vi "Manager.vi"() -> ()   [LabVIEW 2021, in "CIFPluginManager.lvclass"]
uses:
  CIFPluginManager.lvclass
  CIFPluginManager.lvclass/CIFPluginManager.ctl
  <vilib>/gRPC/LabVIEW gRPC Servicer/Servicer/Servicer.lvclass
  gRPC/CIF_Manager_server/RPC Service/Manager/Manager.lvclass
  CIFUtilities/CIFLogs/CIFLogs.lvlib
  gRPC/CIF_Manager_client/RPC Messages/cif_common_Empty.ctl
  gRPC/CIF_Manager_client/CIF_Manager_client.lvlib
  <vilib>/Utility/miscctls.llb/LVMapReplaceAction.ctl
  CIFCore/Grpc/CIFCoreWrapper/CIFCoreWrapper.lvlib
  CIFUtilities/CIFConfigurationFile/CIF Configuration File.lvlib
  gRPC/CIF_Manager_server/RPC Messages/cif_manager_ErrorInfo.ctl
  gRPC/CIF_Manager_server/CIF_Manager_server.lvlib
  gRPC/CIF_Manager_server/RPC Messages/cif_manager_ErrorInfoList.ctl
  gRPC/CIF_Manager_server/RPC Messages/cif_manager_FileData.ctl
  gRPC/CIF_Manager_server/RPC Messages/cif_manager_PluginInfo.ctl
  gRPC/CIF_Manager_server/RPC Messages/cif_manager_PluginInfoArray.ctl
  gRPC/CIF_Manager_server/RPC Messages/cif_manager_PluginType.ctl
  gRPC/CIF_Manager_server/RPC Messages/cif_manager_PluginTypeReply.ctl
  gRPC/CIF_Manager_server/RPC Messages/cif_manager_PluginInfoResponse.ctl
  CIFCore/Common/CIFCoreCommon.lvlib
  CIFCore/Common/Typedef/Errors.ctl
  gRPC/CIF_Manager_server/RPC Messages/cif_manager_TimePair.ctl
  gRPC/CIF_Manager_server/RPC Messages/cif_manager_ClockConversion.ctl
  gRPC/CIF_Manager_server/RPC Messages/cif_manager_ClockConversionArray.ctl
  gRPC/CIF_Manager_server/RPC Messages/cif_manager_SystemStatus.ctl
  gRPC/CIF_Manager_server/RPC Messages/cif_manager_OrchReturn.ctl
  CIFUtilities/Scripting/Orchestration/Python/Python Orchestration.lvlib
  <vilib>/CIF Foundation/CIF Utilities/Time/Time_CIF_U.lvlib
  <vilib>/CIF Foundation/CIF Utilities/Time/Typedef/Timestamp Pair.ctl
  gRPC/CIF_Manager_server/RPC Messages/cif_common_ShortVersion.ctl
  gRPC/CIF_Manager_server/RPC Messages/cif_common_Status.ctl
  gRPC/CIF_Manager_server/RPC Messages/cif_plugincore_MonitorI64.ctl
  gRPC/CIF_Manager_server/RPC Messages/cif_plugincore_MonitorU64.ctl
  gRPC/CIF_Manager_server/RPC Messages/cif_plugincore_MonitorDoubles.ctl
  gRPC/CIF_Manager_server/RPC Messages/cif_plugincore_Error.ctl
  gRPC/CIF_Manager_server/RPC Messages/cif_common_TimingStats.ctl
  gRPC/CIF_Manager_server/RPC Messages/cif_plugincore_FifoStatistics.ctl
  gRPC/CIF_Manager_server/RPC Messages/cif_plugincore_TimingStatistics.ctl
  gRPC/CIF_Manager_server/RPC Messages/cif_plugincore_StatusData_State.ctl
  gRPC/CIF_Manager_server/RPC Messages/cif_plugincore_StatusData.ctl
panel:
  out "error out":errorcluster
  in  "stop":bool
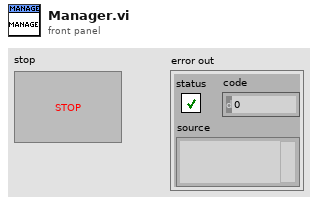
[diagram p1: front panel]
types:
  T1 = typedef "CIF_Manager_client.lvlib/cif_common_Empty.ctl" = cluster{"void":string}
  T2 = typedef "LVMapReplaceAction.ctl" = enum32{"Modify Entry only if found", "Add or Modify Entry", "Delete Entry"}
  T3 = typedef "CIF_Manager_server.lvlib/cif_manager_PluginTypeReply.ctl" = cluster{"plugin_types":T4[]}
  T4 = typedef "CIF_Manager_server.lvlib/cif_manager_PluginType.ctl" = cluster{"plugin_type":string, "plugin_version":T5}
  T5 = typedef "CIF_Manager_server.lvlib/cif_common_ShortVersion.ctl" = cluster{"major":u32, "minor":u32, "fix":u32}
  T6 = typedef "CIF_Manager_server.lvlib/cif_manager_ErrorInfoList.ctl" = cluster{"error_info":T7[]}
  T7 = typedef "CIF_Manager_server.lvlib/cif_manager_ErrorInfo.ctl" = cluster{"error_status":bool, "error_code":i32, "plugin":string, "time":string, "message":string, "location":string}
  T8 = typedef "CIF_Manager_server.lvlib/cif_manager_FileData.ctl" = cluster{"data":string}
  T9 = typedef "CIF_Manager_server.lvlib/cif_manager_PluginInfoArray.ctl" = cluster{"plugin_info":T10[]}
  T10 = typedef "CIF_Manager_server.lvlib/cif_manager_PluginInfo.ctl" = cluster{"plugin_name":string, "plugin_type":string, "grpc_port":i32, "plugin_version":T5, "status":T11}
  T11 = typedef "CIF_Manager_server.lvlib/cif_plugincore_StatusData.ctl" = cluster{"state":T12, "timing_statistics":T13, "fifo_statistics":T15, "error":T16, "monitor_doubles":T17, "monitor_u64s":T18, "monitor_i64s":T19}
  T12 = typedef "CIF_Manager_server.lvlib/cif_plugincore_StatusData_State.ctl" = enum32{"NULL", "CREATING", "LISTENING", "RUNNING", "CLEANINGUP", "DESTROYING"}
  T13 = typedef "CIF_Manager_server.lvlib/cif_plugincore_TimingStatistics.ctl" = cluster{"period":T14, "wake_error":T14, "execute":T14, "housekeep":T14, "idle":T14, "cleanup":T14, "custom_1":T14, "custom_2":T14}
  T14 = typedef "CIF_Manager_server.lvlib/cif_common_TimingStats.ctl" = cluster{"max":i64, "min":i64, "avg":dbl}
  T15 = typedef "CIF_Manager_server.lvlib/cif_plugincore_FifoStatistics.ctl" = cluster{"from_t0":T14, "from_previous_plugin":T14, "output_error":T14}
  T16 = typedef "CIF_Manager_server.lvlib/cif_plugincore_Error.ctl" = cluster{"status":bool, "code":i32}
  T17 = typedef "CIF_Manager_server.lvlib/cif_plugincore_MonitorDoubles.ctl" = cluster{"double_1":dbl, "double_2":dbl, "double_3":dbl, "double_4":dbl}
  T18 = typedef "CIF_Manager_server.lvlib/cif_plugincore_MonitorU64.ctl" = cluster{"u64_1":u64, "u64_2":u64, "u64_3":u64, "u64_4":u64}
  T19 = typedef "CIF_Manager_server.lvlib/cif_plugincore_MonitorI64.ctl" = cluster{"i64_1":i64, "i64_2":i64, "i64_3":i64, "i64_4":i64}
  T20 = typedef "CIFCoreCommon.lvlib/Errors.ctl" = enum16{"Invalid Clock ID", "Long Sleep", "gRPC Server Not Found", "Config Parse", "Timestamp Wrap", "Delayed Execution", "Duplicate Channel", "Missing Channel", "Incorrect Type", "Flatten Error", "Unflatten Data", "Unique Name", "Plugin Not Found", "Plugin Type Not Found", "Plugin Version Not Found", "Manager Not Found", "Numerical Issue", "Time Jump", "Clock ID Match", "Channel Length", "Plugin Connection", "gRPC Server Connection", "PPL Name Match", "Build", "Config Log Parse"}
  T21 = typedef "CIF_Manager_server.lvlib/cif_manager_PluginInfoResponse.ctl" = cluster{"plugin_info":T10, "status":T22}
  T22 = typedef "CIF_Manager_server.lvlib/cif_common_Status.ctl" = cluster{"code":i32, "message":string}
  T23 = typedef "CIF_Manager_server.lvlib/cif_manager_SystemStatus.ctl" = cluster{"clock_conversion_array":T24}
  T24 = typedef "CIF_Manager_server.lvlib/cif_manager_ClockConversionArray.ctl" = cluster{"clock_conversions":T25[]}
  T25 = typedef "CIF_Manager_server.lvlib/cif_manager_ClockConversion.ctl" = cluster{"clock_id":u32, "last_reset":u64, "slope":dbl, "offset_pair":T26, "clock_name":string}
  T26 = typedef "CIF_Manager_server.lvlib/cif_manager_TimePair.ctl" = cluster{"system_time":i64, "external_time":i64}
  T27 = typedef "Time_CIF_U.lvlib/Timestamp Pair.ctl" = cluster{"System Time":i64, "External Time":i64}
  T28 = typedef "CIF_Manager_server.lvlib/cif_manager_OrchReturn.ctl" = cluster{"orchestration_script":string, "status":T22}
  T29 = typedef "grpc-lvsupport-release.lvlib/grpcId.ctl" = u64
  T30 = typedef "CIF_Manager_server.lvlib/cif_manager_PluginConfig.ctl" = cluster{"plugin_type":string, "plugin_name":string, "version":string}
  T31 = typedef "CIF_Manager_client.lvlib/cif_common_Status.ctl" = cluster{"code":i32, "message":string}
  T32 = typedef "CIF_Manager_server.lvlib/cif_manager_RegisterData.ctl" = cluster{"plugin_name":string, "grpc_port":i32, "plugin_version":T5}
  T33 = typedef "CIFPluginManager.lvclass/Plugin Management Data.ctl" = cluster{"vi reference":refnum<vi>, "gRPC ID":T29, "Plugin Type":string, "Unique Name":string, "gRPC Port":i32, "Version":T34, "Load Timestamp":i64, "Unload Timestamp":i64, "Unloading":bool, "Ready for removal":bool, "status":T11}
  T34 = typedef "CIFCoreCommon.lvlib/Version.ctl" = cluster{"Major":i32, "Minor":i32, "Fix":i32, "Build":i32}
  T35 = typedef "CIF_Manager_server.lvlib/cif_manager_PluginName.ctl" = cluster{"plugin_name":string}
  T36 = typedef "CIFPluginManager.lvclass/Discovered Plugin.ctl" = cluster{"Filename":string, "Plugin Type":string, "Qualified name":string, "Version":T34}
  T37 = typedef "CIF_Manager_server.lvlib/cif_manager_QuerySettings.ctl" = cluster{"query_all":bool}
  T38 = typedef "CIFLogs.lvlib/Error Message.ctl" = cluster{"error":bool, "code":i32, "Message":string, "Location":string, "Plugin":string, "Time":string}
  T39 = typedef "CIF_Manager_server.lvlib/cif_manager_PluginStatus.ctl" = cluster{"pluginname":T35, "status":T11}
  T40 = typedef "Time_CIF_U.lvlib/Clock History Map.ctl" = map{u8, T41}
  T41 = typedef "Time_CIF_U.lvlib/Clock History.ctl" = cluster{"System Clock":i64[], "External Clock":i64[], "Last Reset Time":i64, "Slope":dbl[], "slope":dbl, "1/slope":dbl, "Offset Pair":T27, "Name":string}
  T42 = typedef "Time_CIF_U.lvlib/Clock Conversion.ctl" = cluster{"ClockID":u8, "Last Reset":i64, "Offset Pair":T27, "Slope":dbl, "1/Slope":dbl, "Name":string}
  T43 = typedef "CIF_Manager_server.lvlib/cif_manager_ClockUpdate.ctl" = cluster{"clock_id":u32, "timestamp_pair":T26, "reinit":bool, "clock_name":string}
  T44 = typedef "CIF_Manager_server.lvlib/cif_manager_OrchConfig.ctl" = cluster{"start_timestamp":u64, "create_file":bool, "orchestration_language":T45, "filename":string, "default_ip":string}
  T45 = typedef "CIF_Manager_server.lvlib/cif_manager_OrchestrationLanguage.ctl" = enum32{"NULL", "PYTHON"}
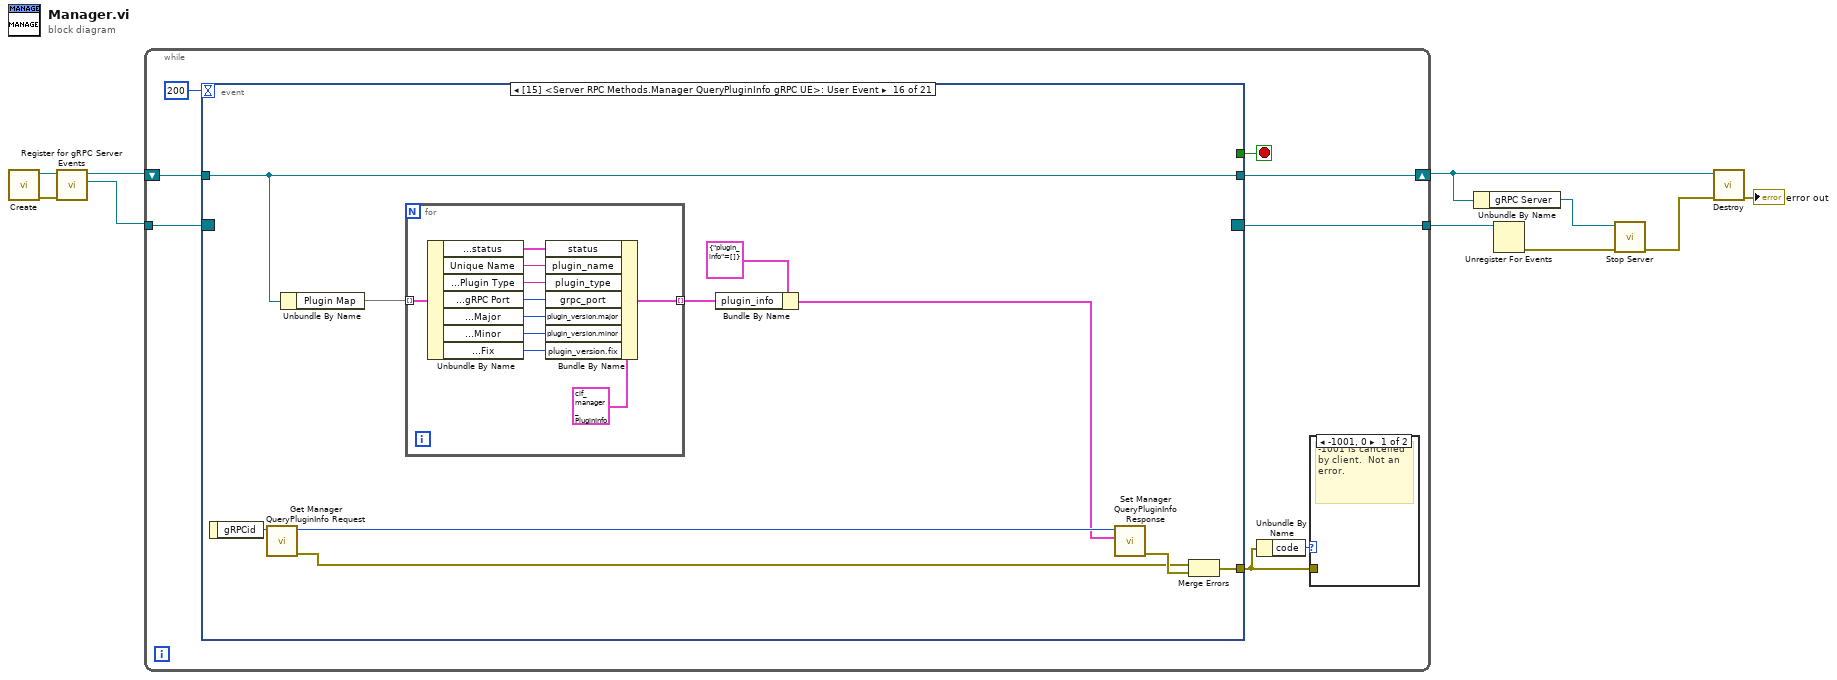
[diagram p0: block diagram]
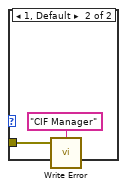
[diagram p2: hidden frame]
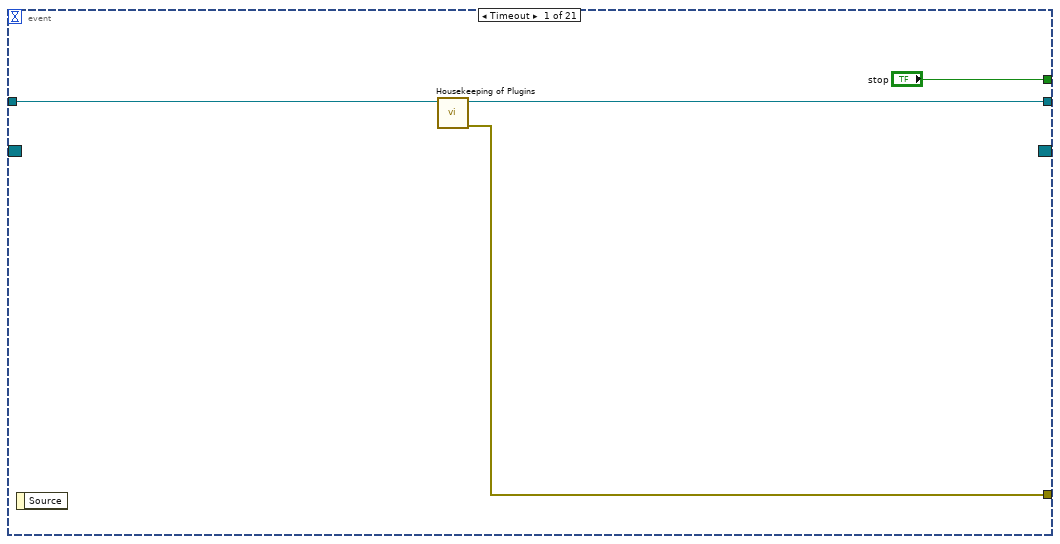
[diagram p3: hidden frame]
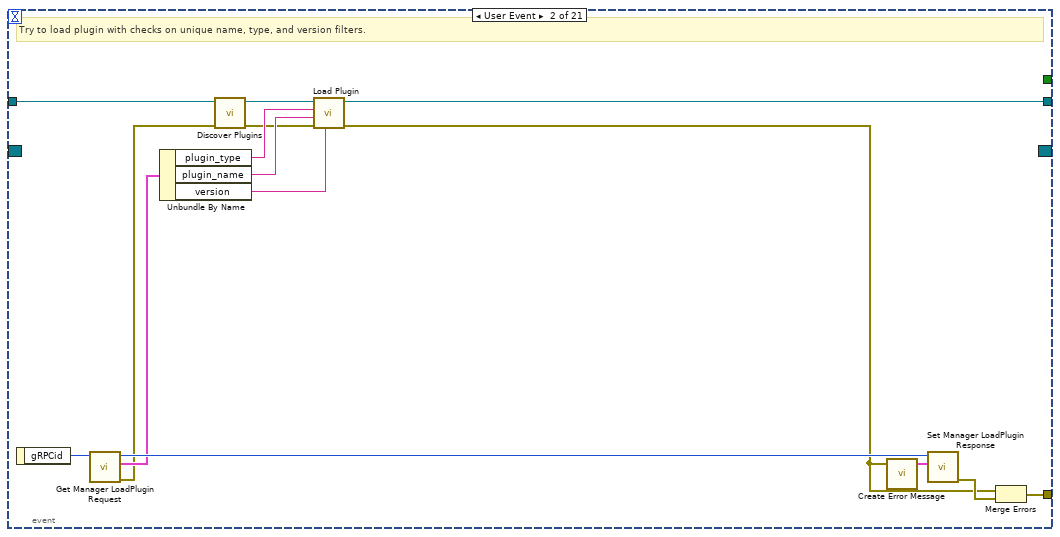
[diagram p4: hidden frame]
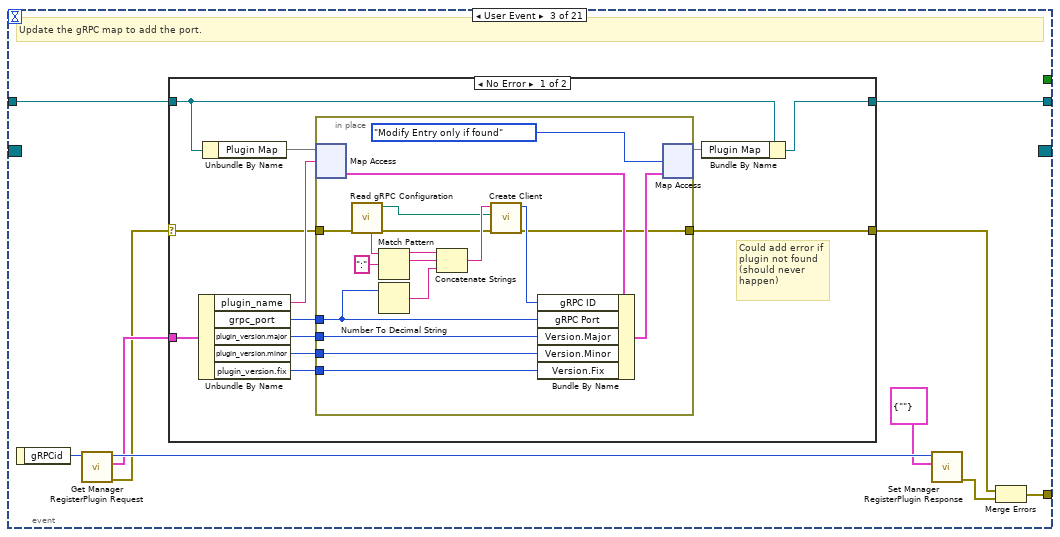
[diagram p5: hidden frame]
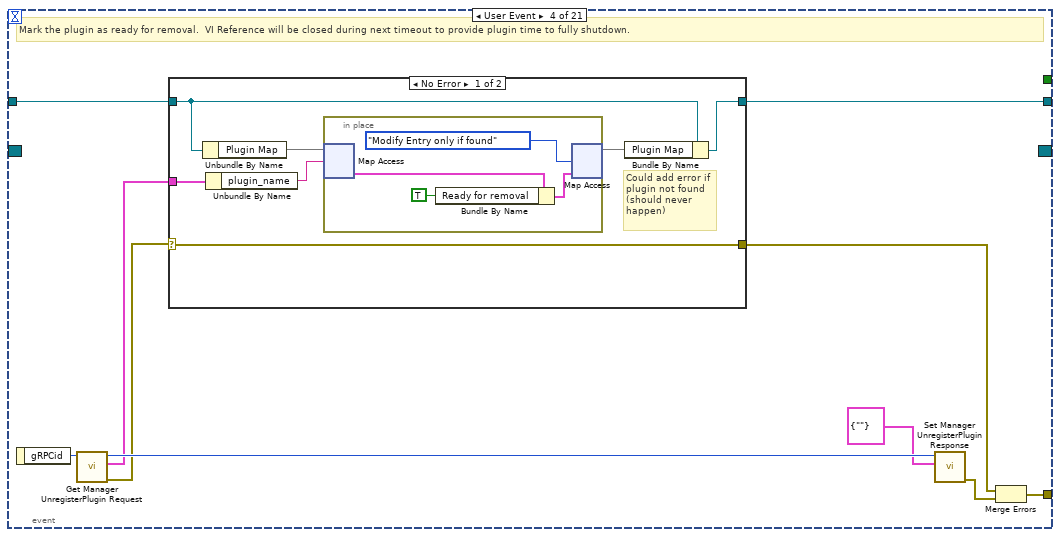
[diagram p7: hidden frame]
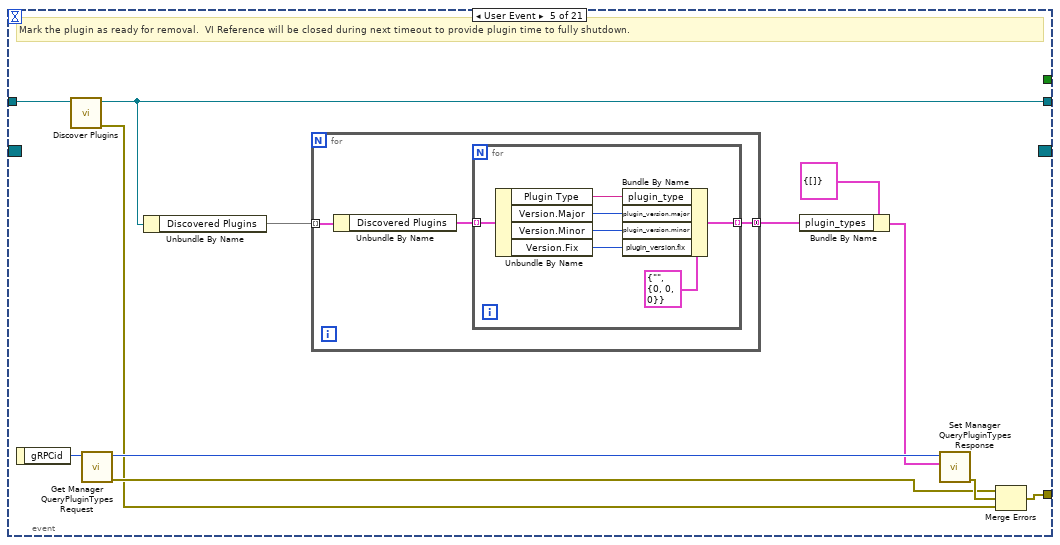
[diagram p9: hidden frame]
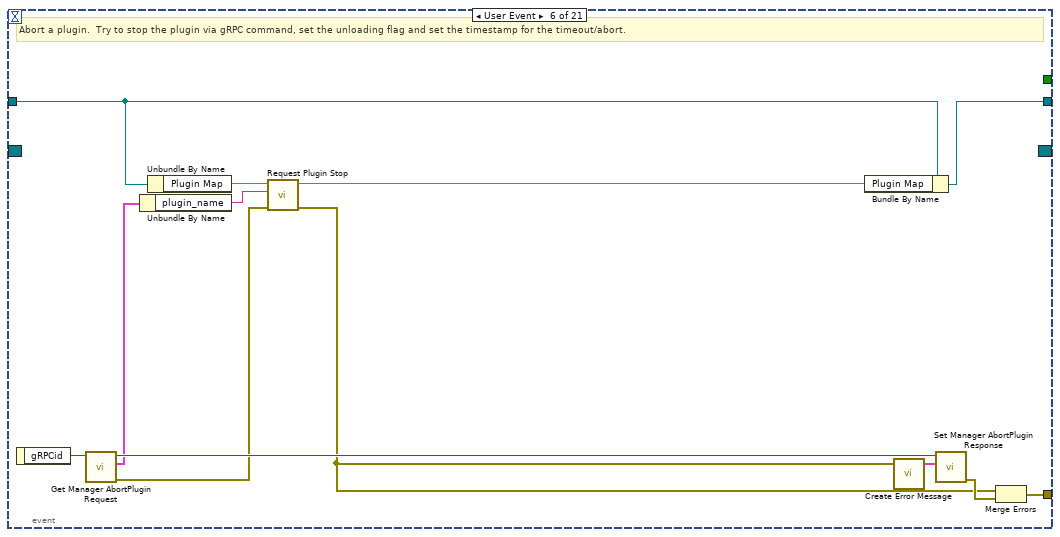
[diagram p10: hidden frame]
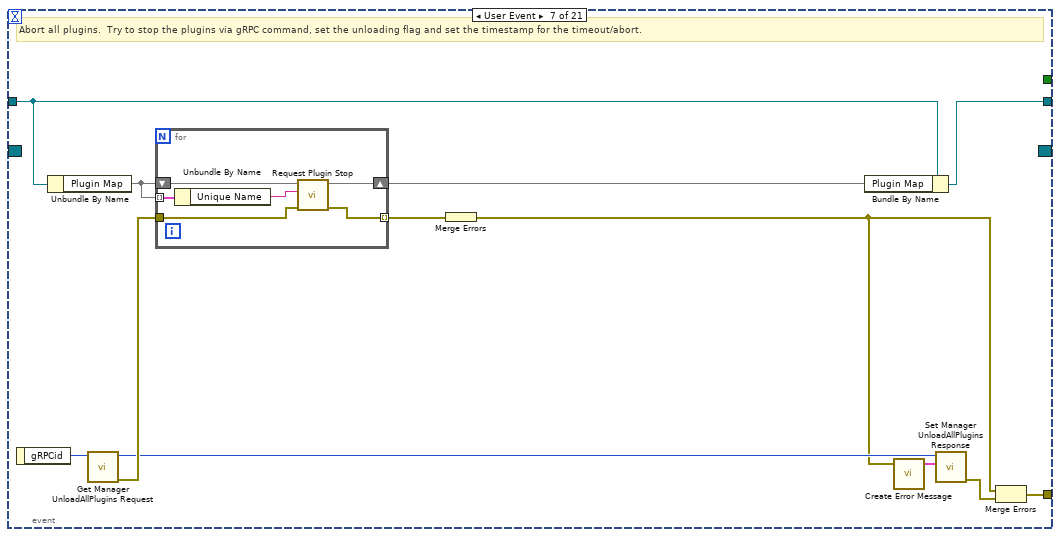
[diagram p11: hidden frame]
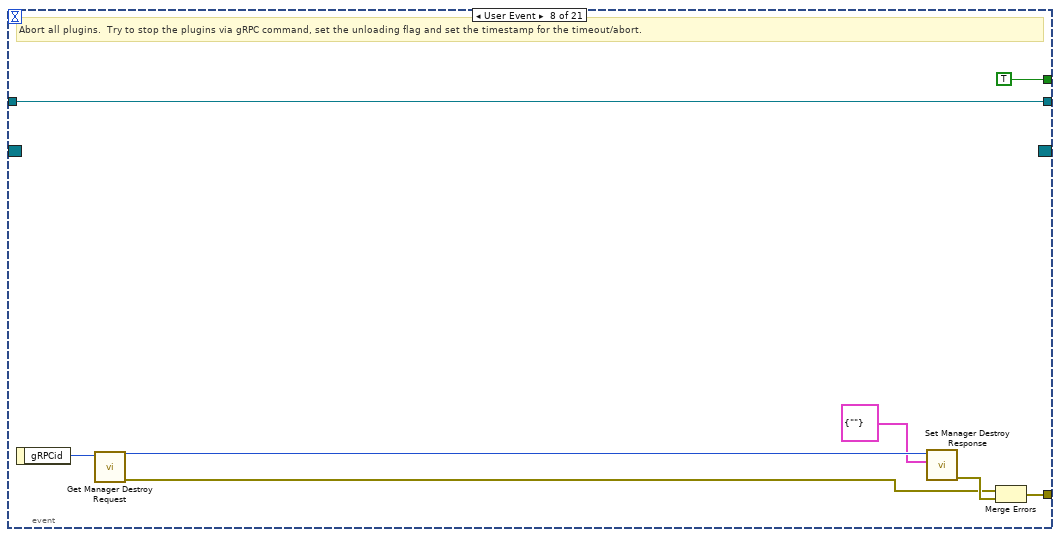
[diagram p12: hidden frame]
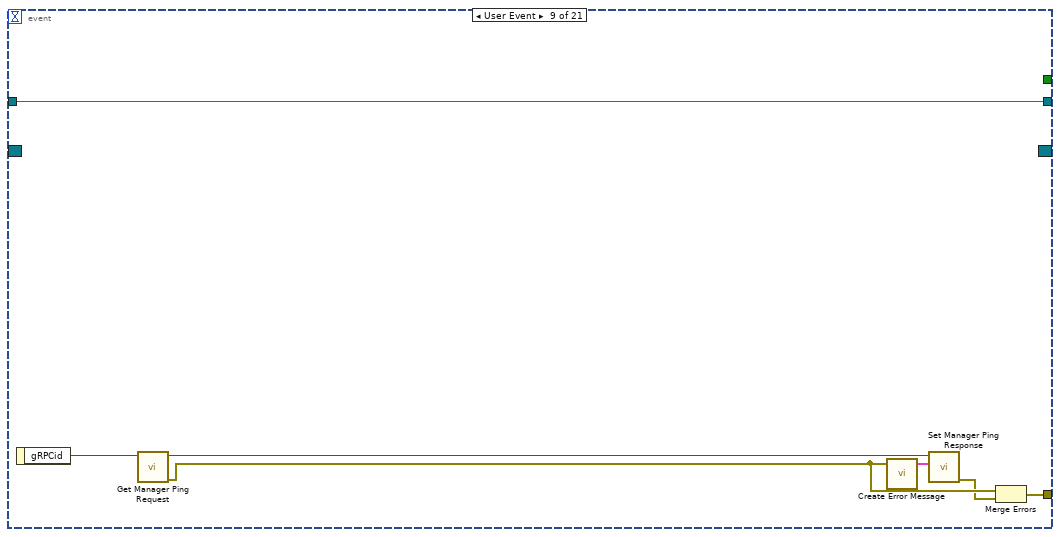
[diagram p13: hidden frame]
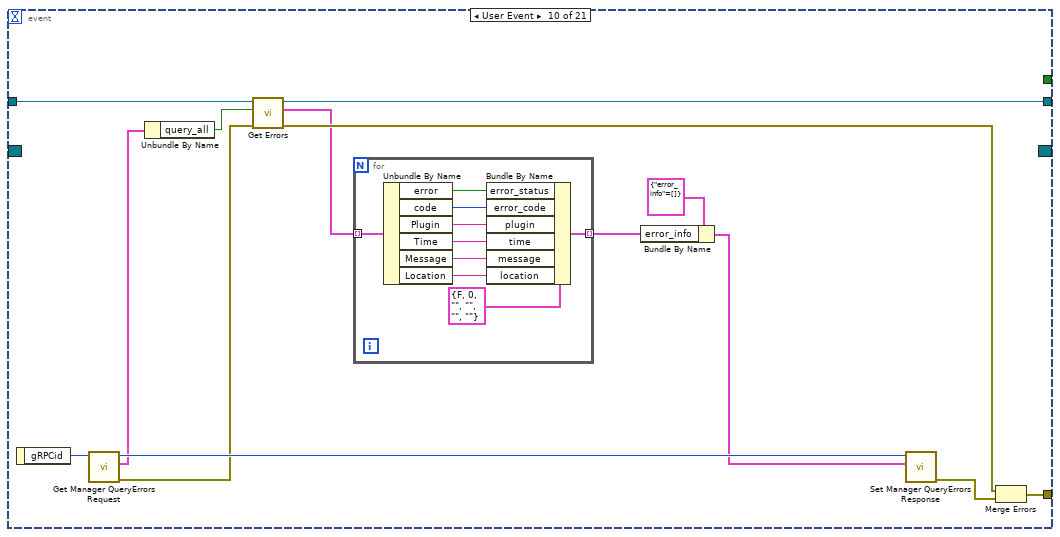
[diagram p14: hidden frame]
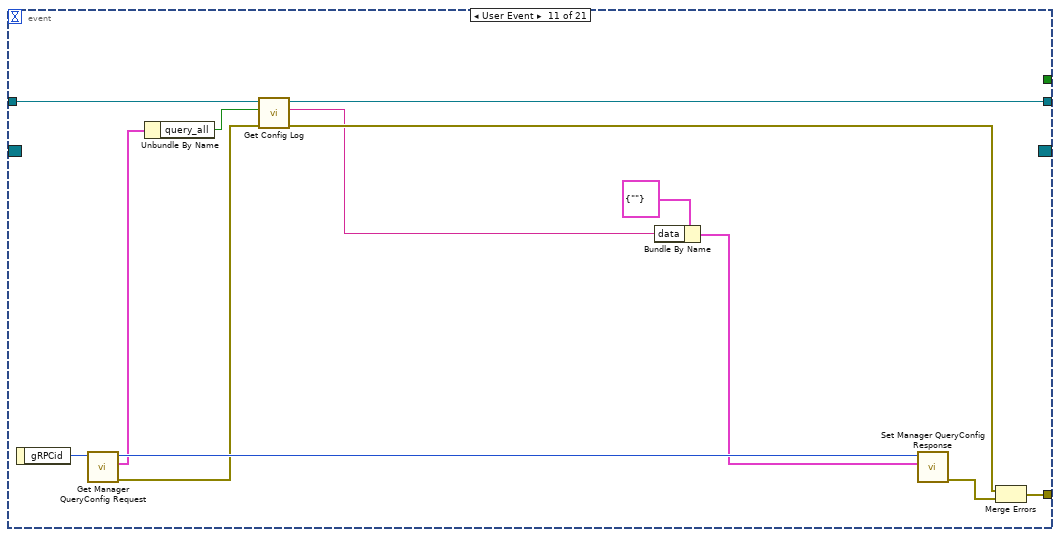
[diagram p15: hidden frame]
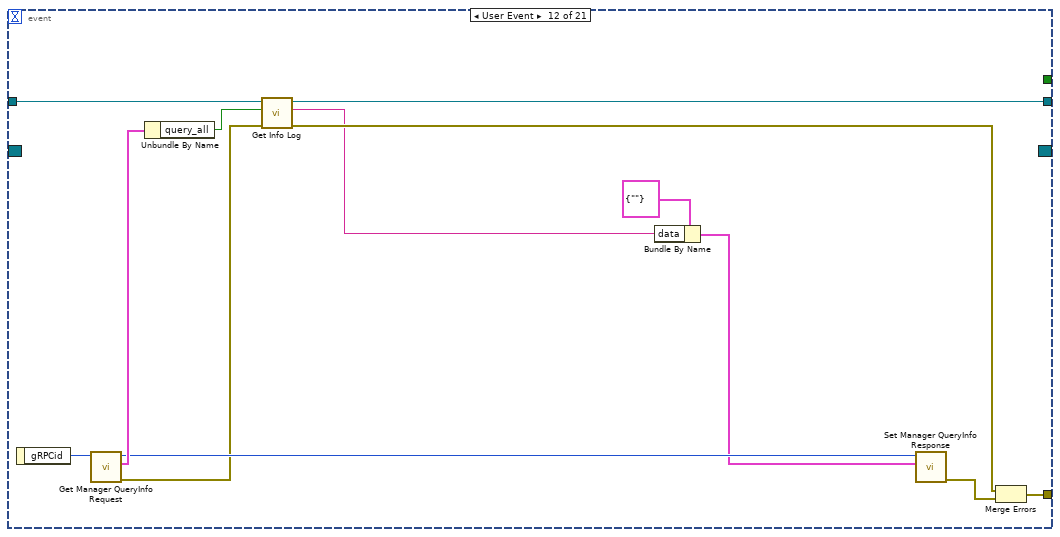
[diagram p16: hidden frame]
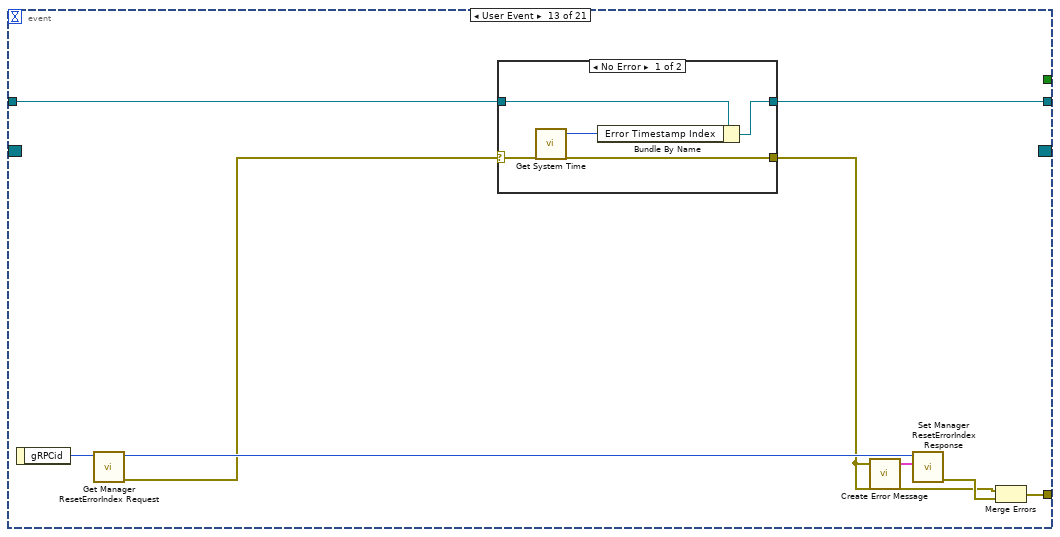
[diagram p17: hidden frame]
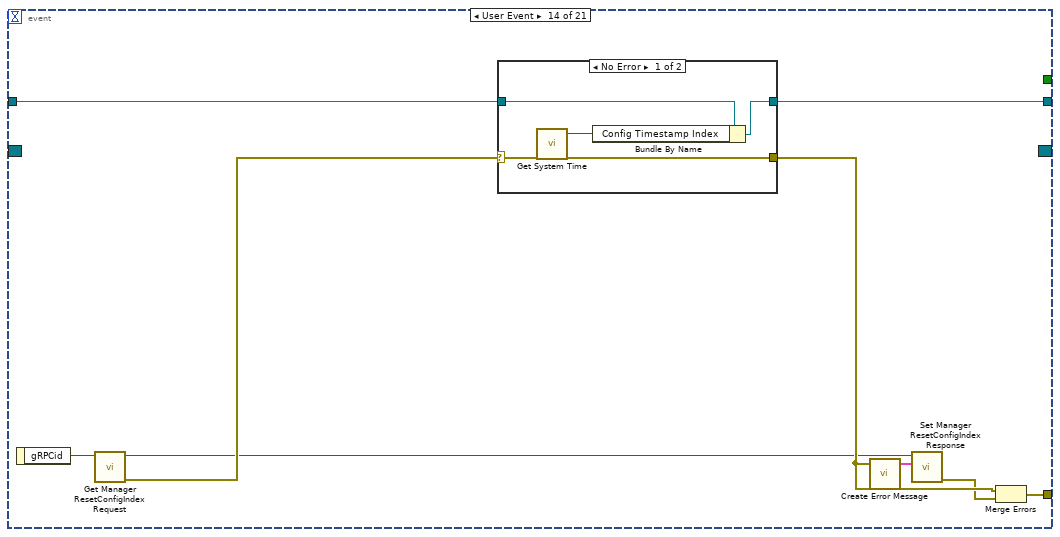
[diagram p19: hidden frame]
diagram:
  n1 = call "Create.vi"() -> ("error out"=w9:errorcluster, "Plugin Manager out"=w10:refnum<class "CIFPluginManager.lvclass">)  [unwired: 10 in]
  n2 = call "Register for gRPC Server Events.vi"("error in (no error)"=w9, "Plugin Manager in"=w10) -> ("Event Registration Refnum"=w8:refnum<event-registration>, "Plugin Manager out"=w7:refnum<class "CIFPluginManager.lvclass">)  [unwired: 7 in, 1 out]
  n3 = while {
    tunnel: w8 -> [w18]
    tunnel: [w14] -> w6
    shift-right: [w15] -> w5
    shift-left: w7 -> [w16]
    stop <- w11 stop-if-true
    n4 = event shown="[15] <Server RPC Methods.Manager QueryPluginInfo gRPC UE>: User Event" {
      selector: w18 -> [_ _ _ _ _ _ _ _ _ _ _ _ _ _ _ _ _ _ _ _ _]
      dyn-events: [_ _ _ _ _ _ _ _ _ _ _ _ _ _ _ _ _ _ _ _ _] -> w14
      timeout: 200 -> [_ _ _ _ _ _ _ _ _ _ _ _ _ _ _ _ _ _ _ _ _]
      tunnel: w16 -> [w24 w28 w43 w90 w107 w133 w150 w160 w166 w182 w201 w214 w224 w244 w259 w275 w307 w318 w352 w381 w400]
      tunnel: [w23 w29 w41 w89 w106 w132 w148 w160 w166 w178 w198 w210 w223 w243 w258 w275 w307 w320 w338 w380 w400] -> w15
      tunnel: [w22 w39 w49 w91 w116 w139 w151 w165 w167 w186 w208 w221 w230 w245 w260 w276 w308 w327 w357 w385 _] -> w12
      tunnel: ["stop" _ _ _ _ _ _ TRUE _ _ _ _ _ _ _ _ _ _ _ _ TRUE] -> w11
      event Timeout {
        n5 = event-data() -> ()  [unwired: 1 in, 1 out]
        n6 = call "Housekeeping of Plugins.vi"("CIFPluginManager in"=w24) -> ("error out"=w22:errorcluster, "CIFPluginManager out"=w23:refnum<class "CIFPluginManager.lvclass">)  [unwired: 9 in]
      }
      event User Event {
        # "Try to load plugin with checks on unique name, type, and version filters."
        n7 = event-data() -> ("gRPCid"=w38:T29)  [unwired: 1 in]
        n8 = call "Get Manager LoadPlugin Request.vi"("gRPCid"=w38) -> ("error out"=w26:errorcluster, "Message Data"=w34:T30, "gRPCid out"=w37:T29)  [unwired: 8 in]
        n9 = Unbundle By Name(w34) -> ("plugin_type"=w33:string, "plugin_name"=w32:string, "version"=w31:string)
        n10 = call "Discover Plugins.vi"("error in (no error)"=w26, "CIFPluginManager in"=w28) -> ("error out"=w25:errorcluster, "CIFPluginManager out"=w27:refnum<class "CIFPluginManager.lvclass">)  [unwired: 8 in]
        n11 = call "Load Plugin.vi"("Version String"=w31, "error in (no error)"=w25, "Unique Name"=w32, "Plugin Type"=w33, "Launcher in"=w27) -> ("error out"=w30:errorcluster, "Launcher out"=w29:refnum<class "CIFPluginManager.lvclass">)  [unwired: 5 in]
        n12 = call "Create Error Message.vi"("error in (no error)"=w30) -> ("Error Message"=w36:T31)  [unwired: 3 in]
        n13 = call "Set Manager LoadPlugin Response.vi"("Message Data"=w36, "gRPCid in"=w37) -> ("error out"=w35:errorcluster)  [unwired: 9 in]
        n14 = Merge Errors(w30, w35) -> (w39:errorcluster)
      }
      event User Event {
        # "Update the gRPC map to add the port."
        n15 = event-data() -> ("gRPCid"=w47:T29)  [unwired: 1 in]
        n16 = call "Get Manager RegisterPlugin Request.vi"("gRPCid"=w47) -> ("error out"=w42:errorcluster, "Message Data"=w44:T32, "gRPCid out"=w48:T29)  [unwired: 8 in]
        n17 = case shown="No Error" w42 {
          selector: w42 -> [w51 w80]
          tunnel: w44 -> [w61 _]
          tunnel: w43 -> [w54 w81]
          tunnel: [w52 w81] -> w41
          tunnel: [w50 w80] -> w40
          frame No Error {
            # "Could add error if plugin not found (should never happen)"
            n18 = Unbundle By Name(w61) -> ("plugin_name"=w59:string, "grpc_port"=w58:i32, "plugin_version.major"=w57:u32, "plugin_version.minor"=w56:u32, "plugin_version.fix"=w55:u32)
            n19 = Unbundle By Name(w54) -> ("Plugin Map"=w60:map{string, T33})
            n20 = in-place {
              in-place-border: w58 -> [w65]
              in-place-border: w57 -> [w76]
              in-place-border: w56 -> [w77]
              in-place-border: w55 -> [w78]
              in-place-border: w51 -> [w63]
              in-place-border: [w62] -> w50
              n21 = in-place-map #1(w60, w59) -> (w79:T33)  [unwired: 1 in, 1 out]
              n22 = call "Read gRPC Configuration.vi"("error in"=w63) -> ("error out"=w67:errorcluster, "Server Certificate File (.crt)"=w72:path, "Local Manager Address"=w68:string)  [unwired: 5 in, 3 out]
              n23 = Match Pattern(string=w68, regular expression=":") -> (before substring=w69:string, match substring=w70:string)  [unwired: 1 in, 2 out]
              n24 = Number To Decimal String(number=w65) -> (decimal integer string=w71:string)  [unwired: 1 in]
              n25 = Concatenate Strings(w69, w70, w71) -> (w73:string)
              n26 = call "Create Client.vi"("error in"=w67, "Server Certificate File (.crt)"=w72, "address"=w73) -> ("error out"=w62:errorcluster, "gRPC ID Out"=w64:T29)  [unwired: 7 in]
              n27 = Bundle By Name(cluster=w79, "gRPC ID"=w64, "gRPC Port"=w65, "Version.Major"=w76, "Version.Minor"=w77, "Version.Fix"=w78) -> (w75:T33)
              n28 = in-place-map #1(w75, LVMapReplaceAction."Modify Entry only if found" ("action")) -> (w53:map{string, T33})  [unwired: 2 out]
            }
            n29 = Bundle By Name(cluster=w54, "Plugin Map"=w53) -> (w52:refnum<class "CIFPluginManager.lvclass">)
          }
          frame Error {
          }
        }
        n30 = call "Set Manager RegisterPlugin Response.vi"("Message Data"=T1 {"void"=""}, "gRPCid in"=w48) -> ("error out"=w46:errorcluster)  [unwired: 9 in]
        n31 = Merge Errors(w40, w46) -> (w49:errorcluster)
      }
      event User Event {
        # "Mark the plugin as ready for removal.  VI Reference will be closed during next timeout to provide plugin time to fully shutdown."
        n32 = event-data() -> ("gRPCid"=w87:T29)  [unwired: 1 in]
        n33 = call "Get Manager UnregisterPlugin Request.vi"("gRPCid"=w87) -> ("error out"=w83:errorcluster, "Message Data"=w82:T35, "gRPCid out"=w86:T29)  [unwired: 8 in]
        n34 = case shown="No Error" w83 {
          selector: w83 -> [w92 w103]
          tunnel: w82 -> [w98 _]
          tunnel: w90 -> [w95 w104]
          tunnel: [w93 w104] -> w89
          tunnel: [w92 w103] -> w88
          frame No Error {
            # "Could add error if plugin not found (should never happen)"
            n35 = Unbundle By Name(w95) -> ("Plugin Map"=w97:map{string, T33})
            n36 = Unbundle By Name(w98) -> ("plugin_name"=w96:string)
            n37 = in-place {
              n38 = in-place-map #2(w97, w96) -> (w101:T33)  [unwired: 1 in, 1 out]
              n39 = Bundle By Name(cluster=w101, "Ready for removal"=TRUE) -> (w100:T33)
              n40 = in-place-map #2(w100, LVMapReplaceAction."Modify Entry only if found" ("action")) -> (w94:map{string, T33})  [unwired: 2 out]
            }
            n41 = Bundle By Name(cluster=w95, "Plugin Map"=w94) -> (w93:refnum<class "CIFPluginManager.lvclass">)
          }
          frame Error {
          }
        }
        n42 = call "Set Manager UnregisterPlugin Response.vi"("Message Data"=T1 {"void"=""}, "gRPCid in"=w86) -> ("error out"=w85:errorcluster)  [unwired: 9 in]
        n43 = Merge Errors(w88, w85) -> (w91:errorcluster)
      }
      event User Event {
        # "Mark the plugin as ready for removal.  VI Reference will be closed during next timeout to provide plugin time to fully shutdown."
        n44 = event-data() -> ("gRPCid"=w115:T29)  [unwired: 1 in]
        n45 = call "Discover Plugins.vi"("CIFPluginManager in"=w107) -> ("error out"=w105:errorcluster, "CIFPluginManager out"=w106:refnum<class "CIFPluginManager.lvclass">)  [unwired: 9 in]
        n46 = call "Get Manager QueryPluginTypes Request.vi"("gRPCid"=w115) -> ("error out"=w109:errorcluster, "gRPCid out"=w114:T29)  [unwired: 8 in, 1 out]
        n47 = Unbundle By Name(w106) -> ("Discovered Plugins"=w112:map{string, T36[]})
        n48 = for {
          tunnel: w112 -> [w119] mode=indexing
          tunnel: [w117] -> w110 mode=concatenating
          n49 = Unbundle By Name(w119) -> ("Discovered Plugins"=w118:T36[])
          n50 = for {
            tunnel: w118 -> [w126] mode=indexing
            tunnel: [w120] -> w117 mode=indexing
            n51 = Unbundle By Name(w126) -> ("Plugin Type"=w121:string, "Version.Major"=w122:i32, "Version.Minor"=w123:i32, "Version.Fix"=w124:i32)
            n52 = Bundle By Name(cluster=T4 {"plugin_type"="", "plugin_version"={"major"=0, "minor"=0, "fix"=0}} ("cif_manager_PluginType"), "plugin_type"=w121, "plugin_version.major"=w122, "plugin_version.minor"=w123, "plugin_version.fix"=w124) -> (w120:T4)
          }
        }
        n53 = Bundle By Name(cluster=T3 {"plugin_types"=[]} ("Message Data"), "plugin_types"=w110) -> (w108:T3)
        n54 = call "Set Manager QueryPluginTypes Response.vi"("Message Data"=w108, "gRPCid in"=w114) -> ("error out"=w113:errorcluster)  [unwired: 9 in]
        n55 = Merge Errors(w109, w113, w105) -> (w116:errorcluster)
      }
      event User Event {
        # "Abort a plugin.  Try to stop the plugin via gRPC command, set the unloading flag and set the timestamp for the timeout/abort."
        n56 = event-data() -> ("gRPCid"=w138:T29)  [unwired: 1 in]
        n57 = call "Get Manager AbortPlugin Request.vi"("gRPCid"=w138) -> ("error out"=w130:errorcluster, "Message Data"=w135:T35, "gRPCid out"=w137:T29)  [unwired: 8 in]
        n58 = Unbundle By Name(w135) -> ("plugin_name"=w129:string)
        n59 = Unbundle By Name(w133) -> ("Plugin Map"=w131:map{string, T33})
        n60 = call "Request Plugin Stop.vi"("error in (no error)"=w130, "Unique Name"=w129, "Plugin Map in"=w131) -> ("error out"=w127:errorcluster, "Plugin Map out"=w128:map{string, T33})  [unwired: 7 in]
        n61 = Bundle By Name(cluster=w133, "Plugin Map"=w128) -> (w132:refnum<class "CIFPluginManager.lvclass">)
        n62 = call "Create Error Message.vi"("error in (no error)"=w127) -> ("Error Message"=w134:T31)  [unwired: 3 in]
        n63 = call "Set Manager AbortPlugin Response.vi"("Message Data"=w134, "gRPCid in"=w137) -> ("error out"=w136:errorcluster)  [unwired: 9 in]
        n64 = Merge Errors(w127, w136) -> (w139:errorcluster)
      }
      event User Event {
        # "Abort all plugins.  Try to stop the plugins via gRPC command, set the unloading flag and set the timestamp for the timeout/abort."
        n65 = event-data() -> ("gRPCid"=w146:T29)  [unwired: 1 in]
        n66 = Unbundle By Name(w150) -> ("Plugin Map"=w144:map{string, T33})
        n67 = call "Get Manager UnloadAllPlugins Request.vi"("gRPCid"=w146) -> ("error out"=w143:errorcluster, "gRPCid out"=w142:T29)  [unwired: 8 in, 1 out]
        n68 = for {
          shift-right: [w153] -> w149
          shift-left: w144 -> [w156]
          tunnel: w143 -> [w155]
          tunnel: [w154] -> w147 mode=indexing
          tunnel: w144 -> [w157] mode=indexing
          n69 = Unbundle By Name(w157) -> ("Unique Name"=w152:string)
          n70 = call "Request Plugin Stop.vi"("error in (no error)"=w155, "Unique Name"=w152, "Plugin Map in"=w156) -> ("error out"=w154:errorcluster, "Plugin Map out"=w153:map{string, T33})  [unwired: 7 in]
        }
        n71 = Merge Errors(w147) -> (w140:errorcluster)
        n72 = Bundle By Name(cluster=w150, "Plugin Map"=w149) -> (w148:refnum<class "CIFPluginManager.lvclass">)
        n73 = call "Create Error Message.vi"("error in (no error)"=w140) -> ("Error Message"=w145:T31)  [unwired: 3 in]
        n74 = call "Set Manager UnloadAllPlugins Response.vi"("Message Data"=w145, "gRPCid in"=w142) -> ("error out"=w141:errorcluster)  [unwired: 9 in]
        n75 = Merge Errors(w140, w141) -> (w151:errorcluster)
      }
      event User Event {
        # "Abort all plugins.  Try to stop the plugins via gRPC command, set the unloading flag and set the timestamp for the timeout/abort."
        n76 = event-data() -> ("gRPCid"=w164:T29)  [unwired: 1 in]
        n77 = call "Get Manager Destroy Request.vi"("gRPCid"=w164) -> ("error out"=w158:errorcluster, "gRPCid out"=w163:T29)  [unwired: 8 in, 1 out]
        n78 = call "Set Manager Destroy Response.vi"("Message Data"=T1 {"void"=""}, "gRPCid in"=w163) -> ("error out"=w162:errorcluster)  [unwired: 9 in]
        n79 = Merge Errors(w158, w162) -> (w165:errorcluster)
      }
      event User Event {
        n80 = event-data() -> ("gRPCid"=w172:T29)  [unwired: 1 in]
        n81 = call "Get Manager Ping Request.vi"("gRPCid"=w172) -> ("error out"=w169:errorcluster, "gRPCid out"=w171:T29)  [unwired: 8 in, 1 out]
        n82 = call "Create Error Message.vi"("error in (no error)"=w169) -> ("Error Message"=w170:T31)  [unwired: 3 in]
        n83 = call "Set Manager Ping Response.vi"("Message Data"=w170, "gRPCid in"=w171) -> ("error out"=w168:errorcluster)  [unwired: 9 in]
        n84 = Merge Errors(w169, w168) -> (w167:errorcluster)
      }
      event User Event {
        n85 = event-data() -> ("gRPCid"=w185:T29)  [unwired: 1 in]
        n86 = call "Get Manager QueryErrors Request.vi"("gRPCid"=w185) -> ("error out"=w181:errorcluster, "Message Data"=w180:T37, "gRPCid out"=w184:T29)  [unwired: 8 in]
        n87 = Unbundle By Name(w180) -> ("query_all"=w179:bool)
        n88 = call "Get Errors.vi"("error in (no error)"=w181, "Parse All"=w179, "Plugin Manager in"=w182) -> ("error out"=w177:errorcluster, "Errors"=w176:T38[], "Plugin Manager out"=w178:refnum<class "CIFPluginManager.lvclass">)  [unwired: 6 in]
        n89 = for {
          tunnel: w176 -> [w195] mode=indexing
          tunnel: [w187] -> w174 mode=indexing
          n90 = Unbundle By Name(w195) -> ("error"=w193:bool, "code"=w192:i32, "Plugin"=w191:string, "Time"=w190:string, "Message"=w189:string, "Location"=w188:string)
          n91 = Bundle By Name(cluster=T7 {"error_status"=FALSE, "error_code"=0, "plugin"="", "time"="", "message"="", "location"=""} ("cif_manager_ErrorInfo"), "error_status"=w193, "error_code"=w192, "plugin"=w191, "time"=w190, "message"=w189, "location"=w188) -> (w187:T7)
        }
        n92 = Bundle By Name(cluster=T6 {"error_info"=[]} ("Message Data"), "error_info"=w174) -> (w173:T6)
        n93 = call "Set Manager QueryErrors Response.vi"("Message Data"=w173, "gRPCid in"=w184) -> ("error out"=w183:errorcluster)  [unwired: 9 in]
        n94 = Merge Errors(w177, w183) -> (w186:errorcluster)
      }
      event User Event {
        n95 = event-data() -> ("gRPCid"=w206:T29)  [unwired: 1 in]
        n96 = call "Get Manager QueryConfig Request.vi"("gRPCid"=w206) -> ("error out"=w200:errorcluster, "Message Data"=w205:T37, "gRPCid out"=w207:T29)  [unwired: 8 in]
        n97 = Unbundle By Name(w205) -> ("query_all"=w199:bool)
        n98 = call "Get Config Log.vi"("error in (no error)"=w200, "Parse All"=w199, "Plugin Manager in"=w201) -> ("error out"=w197:errorcluster, "Filtered Config Entries"=w196:string, "Plugin Manager out"=w198:refnum<class "CIFPluginManager.lvclass">)  [unwired: 6 in]
        n99 = Bundle By Name(cluster=T8 {"data"=""} ("Message Data"), "data"=w196) -> (w202:T8)
        n100 = call "Set Manager QueryConfig Response.vi"("Message Data"=w202, "gRPCid in"=w207) -> ("error out"=w204:errorcluster)  [unwired: 9 in]
        n101 = Merge Errors(w197, w204) -> (w208:errorcluster)
      }
      event User Event {
        n102 = event-data() -> ("gRPCid"=w219:T29)  [unwired: 1 in]
        n103 = call "Get Manager QueryInfo Request.vi"("gRPCid"=w219) -> ("error out"=w212:errorcluster, "Message Data"=w218:T37, "gRPCid out"=w217:T29)  [unwired: 8 in]
        n104 = Unbundle By Name(w218) -> ("query_all"=w213:bool)
        n105 = call "Get Info Log.vi"("error in (no error)"=w212, "Parse All"=w213, "Plugin Manager in"=w214) -> ("error out"=w211:errorcluster, "Filtered Info Entries"=w209:string, "Plugin Manager out"=w210:refnum<class "CIFPluginManager.lvclass">)  [unwired: 6 in]
        n106 = Bundle By Name(cluster=T8 {"data"=""} ("Message Data"), "data"=w209) -> (w215:T8)
        n107 = call "Set Manager QueryInfo Response.vi"("Message Data"=w215, "gRPCid in"=w217) -> ("error out"=w216:errorcluster)  [unwired: 9 in]
        n108 = Merge Errors(w211, w216) -> (w221:errorcluster)
      }
      event User Event {
        n109 = event-data() -> ("gRPCid"=w229:T29)  [unwired: 1 in]
        n110 = call "Get Manager ResetErrorIndex Request.vi"("gRPCid"=w229) -> ("error out"=w225:errorcluster, "gRPCid out"=w228:T29)  [unwired: 8 in, 1 out]
        n111 = case shown="No Error" w225 {
          selector: w225 -> [w231 w235]
          tunnel: w224 -> [w234 w236]
          tunnel: [w233 w236] -> w223
          tunnel: [w231 w235] -> w222
          frame No Error {
            n112 = call <vilib>:"Get System Time.vi"() -> ("Time (ns)"=w232:i64)  [unwired: 5 in]
            n113 = Bundle By Name(cluster=w234, "Error Timestamp Index"=w232) -> (w233:refnum<class "CIFPluginManager.lvclass">)
          }
          frame Error {
          }
        }
        n114 = call "Create Error Message.vi"("error in (no error)"=w222) -> ("Error Message"=w226:T31)  [unwired: 3 in]
        n115 = call "Set Manager ResetErrorIndex Response.vi"("Message Data"=w226, "gRPCid in"=w228) -> ("error out"=w227:errorcluster)  [unwired: 9 in]
        n116 = Merge Errors(w222, w227) -> (w230:errorcluster)
      }
      event User Event {
        n117 = event-data() -> ("gRPCid"=w241:T29)  [unwired: 1 in]
        n118 = call "Get Manager ResetConfigIndex Request.vi"("gRPCid"=w241) -> ("error out"=w240:errorcluster, "gRPCid out"=w239:T29)  [unwired: 8 in, 1 out]
        n119 = case shown="No Error" w240 {
          selector: w240 -> [w246 w250]
          tunnel: w244 -> [w249 w251]
          tunnel: [w248 w251] -> w243
          tunnel: [w246 w250] -> w242
          frame No Error {
            n120 = call <vilib>:"Get System Time.vi"() -> ("Time (ns)"=w247:i64)  [unwired: 5 in]
            n121 = Bundle By Name(cluster=w249, "Config Timestamp Index"=w247) -> (w248:refnum<class "CIFPluginManager.lvclass">)
          }
          frame Error {
          }
        }
        n122 = call "Create Error Message.vi"("error in (no error)"=w242) -> ("Error Message"=w237:T31)  [unwired: 3 in]
        n123 = call "Set Manager ResetConfigIndex Response.vi"("Message Data"=w237, "gRPCid in"=w239) -> ("error out"=w238:errorcluster)  [unwired: 9 in]
        n124 = Merge Errors(w242, w238) -> (w245:errorcluster)
      }
      event User Event {
        n125 = event-data() -> ("gRPCid"=w256:T29)  [unwired: 1 in]
        n126 = call "Get Manager ResetInfoIndex Request.vi"("gRPCid"=w256) -> ("error out"=w255:errorcluster, "gRPCid out"=w252:T29)  [unwired: 8 in, 1 out]
        n127 = case shown="No Error" w255 {
          selector: w255 -> [w261 w265]
          tunnel: w259 -> [w264 w266]
          tunnel: [w263 w266] -> w258
          tunnel: [w261 w265] -> w257
          frame No Error {
            n128 = call <vilib>:"Get System Time.vi"() -> ("Time (ns)"=w262:i64)  [unwired: 5 in]
            n129 = Bundle By Name(cluster=w264, "Info Timestamp Index"=w262) -> (w263:refnum<class "CIFPluginManager.lvclass">)
          }
          frame Error {
          }
        }
        n130 = call "Create Error Message.vi"("error in (no error)"=w257) -> ("Error Message"=w253:T31)  [unwired: 3 in]
        n131 = call "Set Manager ResetInfoIndex Response.vi"("Message Data"=w253, "gRPCid in"=w252) -> ("error out"=w254:errorcluster)  [unwired: 9 in]
        n132 = Merge Errors(w257, w254) -> (w260:errorcluster)
      }
      event User Event {
        n133 = event-data() -> ("gRPCid"=w274:T29)  [unwired: 1 in]
        n134 = call "Get Manager QueryPluginInfo Request.vi"("gRPCid"=w274) -> ("error out"=w270:errorcluster, "gRPCid out"=w273:T29)  [unwired: 8 in, 1 out]
        n135 = Unbundle By Name(w275) -> ("Plugin Map"=w271:map{string, T33})
        n136 = for {
          tunnel: w271 -> [w286] mode=indexing
          tunnel: [w281] -> w268 mode=indexing
          n137 = Unbundle By Name(w286) -> ("Plugin Management Data.status"=w277:T11, "Unique Name"=w284:string, "Plugin Management Data.Plugin Type"=w283:string, "Plugin Management Data.gRPC Port"=w282:i32, "Plugin Management Data.Version.Major"=w278:i32, "Plugin Management Data.Version.Minor"=w279:i32, "Plugin Management Data.Version.Fix"=w280:i32)
          n138 = Bundle By Name(cluster=T10 {"plugin_name"="", "plugin_type"="", "grpc_port"=0, "plugin_version"={"major"=0, "minor"=0, "fix"=0}, "status"={"state"=enum."NULL", "timing_statistics"={"period"={"max"=0, "min"=0, "avg"=0.0}, "wake_error"={"max"=0, "min"=0, "avg"=0.0}, "execute"={"max"=0, "min"=0, "avg"=0.0}, "housekeep"={"max"=0, "min"=0, "avg"=0.0}, "idle"={"max"=0, "min"=0, "avg"=0.0}, "cleanup"={"max"=0, "min"=0, "avg"=0.0}, "custom_1"={"max"=0, "min"=0, "avg"=0.0}, "custom_2"={"max"=0, "min"=0, "avg"=0.0}}, "fifo_statistics"={"from_t0"={"max"=0, "min"=0, "avg"=0.0}, "from_previous_plugin"={"max"=0, "min"=0, "avg"=0.0}, "output_error"={"max"=0, "min"=0, "avg"=0.0}}, "error"={"status"=FALSE, "code"=0}, "monitor_doubles"={"double_1"=0.0, "double_2"=0.0, "double_3"=0.0, "double_4"=0.0}, "monitor_u64s"={"u64_1"=0, "u64_2"=0, "u64_3"=0, "u64_4"=0}, "monitor_i64s"={"i64_1"=0, "i64_2"=0, "i64_3"=0, "i64_4"=0}}} ("cif_manager_PluginInfo"), "status"=w277, "plugin_name"=w284, "plugin_type"=w283, "grpc_port"=w282, "plugin_version.major"=w278, "plugin_version.minor"=w279, "plugin_version.fix"=w280) -> (w281:T10)
        }
        n139 = Bundle By Name(cluster=T9 {"plugin_info"=[]} ("Message Data"), "plugin_info"=w268) -> (w267:T9)
        n140 = call "Set Manager QueryPluginInfo Response.vi"("Message Data"=w267, "gRPCid in"=w273) -> ("error out"=w272:errorcluster)  [unwired: 9 in]
        n141 = Merge Errors(w270, w272) -> (w276:errorcluster)
      }
      event User Event {
        n142 = event-data() -> ("gRPCid"=w306:T29)  [unwired: 1 in]
        n143 = call "Get Manager QueryPlugin Request.vi"("gRPCid"=w306) -> ("error out"=w290:errorcluster, "Message Data"=w299:T35, "gRPCid out"=w305:T29)  [unwired: 8 in]
        n144 = Unbundle By Name(w299) -> ("plugin_name"=w288:string)
        n145 = Unbundle By Name(w307) -> ("Plugin Map"=w300:map{string, T33})
        n146 = Look In Map(map=w300, key=w288) -> (key not found?=w287:bool, value=w298:T33)  [unwired: 1 in]
        n147 = call "Add Error.vi"("error in (no error)"=w290, "String to Append"=w288, "Error"=Errors."Plugin Not Found", "Insert Error"=w287) -> ("error out"=w289:errorcluster)  [unwired: 7 in]
        n148 = Unbundle By Name(w298) -> ("Unique Name"=w303:string, "Plugin Type"=w302:string, "gRPC Port"=w301:i32, "Version.Major"=w296:i32, "Version.Minor"=w294:i32, "Version.Fix"=w295:i32)
        n149 = call "Create Error Message.vi"("error in (no error)"=w289) -> ("Error Message"=w293:T31)  [unwired: 3 in]
        n150 = Bundle By Name(cluster=T21 {"plugin_info"={"plugin_name"="", "plugin_type"="", "grpc_port"=0, "plugin_version"={"major"=0, "minor"=0, "fix"=0}, "status"={"state"=enum."NULL", "timing_statistics"={"period"={"max"=0, "min"=0, "avg"=0.0}, "wake_error"={"max"=0, "min"=0, "avg"=0.0}, "execute"={"max"=0, "min"=0, "avg"=0.0}, "housekeep"={"max"=0, "min"=0, "avg"=0.0}, "idle"={"max"=0, "min"=0, "avg"=0.0}, "cleanup"={"max"=0, "min"=0, "avg"=0.0}, "custom_1"={"max"=0, "min"=0, "avg"=0.0}, "custom_2"={"max"=0, "min"=0, "avg"=0.0}}, "fifo_statistics"={"from_t0"={"max"=0, "min"=0, "avg"=0.0}, "from_previous_plugin"={"max"=0, "min"=0, "avg"=0.0}, "output_error"={"max"=0, "min"=0, "avg"=0.0}}, "error"={"status"=FALSE, "code"=0}, "monitor_doubles"={"double_1"=0.0, "double_2"=0.0, "double_3"=0.0, "double_4"=0.0}, "monitor_u64s"={"u64_1"=0, "u64_2"=0, "u64_3"=0, "u64_4"=0}, "monitor_i64s"={"i64_1"=0, "i64_2"=0, "i64_3"=0, "i64_4"=0}}}, "status"={"code"=0, "message"=""}} ("Message Data"), "plugin_info.plugin_name"=w303, "plugin_info.plugin_type"=w302, "plugin_info.grpc_port"=w301, "plugin_info.plugin_version.major"=w296, "plugin_info.plugin_version.minor"=w294, "plugin_info.plugin_version.fix"=w295, "status"=w293) -> (w292:T21)
        n151 = call "Set Manager QueryPlugin Response.vi"("Message Data"=w292, "gRPCid in"=w305) -> ("error out"=w304:errorcluster)  [unwired: 9 in]
        n152 = Merge Errors(w289, w304) -> (w308:errorcluster)
      }
      event User Event {
        n153 = event-data() -> ("gRPCid"=w326:T29)  [unwired: 1 in]
        n154 = call "Get Manager QuerySystemStatus Request.vi"("gRPCid"=w326) -> ("error out"=w315:errorcluster, "Message Data"=w319:T39, "gRPCid out"=w325:T29)  [unwired: 8 in]
        n155 = Unbundle By Name(w319) -> ("pluginname.plugin_name"=w317:string, "status"=w316:T11)
        n156 = call "Update Plugin Status.vi"("error in (no error)"=w315, "Status"=w316, "Plugin Name"=w317, "Launcher in"=w318) -> ("error out"=w311:errorcluster, "Launcher out"=w314:refnum<class "CIFPluginManager.lvclass">)  [unwired: 6 in]
        n157 = Unbundle By Name(w314) -> ("Clock History Map"=w313:T40)
        n158 = call <vilib>:"Clock Map to Clock Array.vi"("error in (no error)"=w311, "Clock History Map in"=w313) -> ("error out"=w310:errorcluster, "Clock Conversion Array"=w309:T42[], "Clock History Map out"=w312:T40)  [unwired: 7 in]
        n159 = for {
          tunnel: w309 -> [w336] mode=indexing
          tunnel: [w328] -> w322 mode=indexing
          n160 = Unbundle By Name(w336) -> ("ClockID"=w335:u8, "Last Reset"=w329:i64, "Offset Pair.System Time"=w330:i64, "Offset Pair.External Time"=w331:i64, "Slope"=w332:dbl, "Name"=w333:string)
          n161 = To Unsigned Long Integer(number=w335) -> (unsigned 32bit integer=w334:u32)
          n162 = Bundle By Name(cluster=T25 {"clock_id"=0, "last_reset"=0, "slope"=0.0, "offset_pair"={"system_time"=0, "external_time"=0}, "clock_name"=""} ("cif_manager_ClockConversion"), "clock_id"=w334, "last_reset"=w329, "offset_pair.system_time"=w330, "offset_pair.external_time"=w331, "slope"=w332, "clock_name"=w333) -> (w328:T25)
        }
        n163 = Bundle By Name(cluster=w314, "Clock History Map"=w312) -> (w320:refnum<class "CIFPluginManager.lvclass">)
        n164 = Bundle By Name(cluster=T23 {"clock_conversion_array"={"clock_conversions"=[]}} ("Message Data"), "clock_conversion_array.clock_conversions"=w322) -> (w321:T23)
        n165 = call "Set Manager QuerySystemStatus Response.vi"("Message Data"=w321, "gRPCid in"=w325) -> ("error out"=w324:errorcluster)  [unwired: 9 in]
        n166 = Merge Errors(w310, w324) -> (w327:errorcluster)
      }
      event User Event {
        n167 = event-data() -> ("gRPCid"=w356:T29)  [unwired: 1 in]
        n168 = call "Get Manager UpdateClock Request.vi"("gRPCid"=w356) -> ("error out"=w348:errorcluster, "Message Data"=w347:T43, "gRPCid out"=w355:T29)  [unwired: 8 in]
        n169 = Unbundle By Name(w352) -> ("Clock History Map"=w353:T40)
        n170 = Unbundle By Name(w347) -> ("timestamp_pair.system_time"=w341:i64, "timestamp_pair.external_time"=w340:i64, "reinit"=w343:bool, "clock_id"=w346:u32, "clock_name"=w345:string)
        n171 = Bundle By Name(cluster=T27 {"System Time"=0, "External Time"=0} ("Timestamp Pair"), "System Time"=w341, "External Time"=w340) -> (w339:T27)
        n172 = To Unsigned Byte Integer(number=w346) -> (unsigned 8bit integer=w344:u8)
        n173 = call <vilib>:"Update Clock Map.vi"("Name"=w345, "Reset"=w343, "error in (no error)"=w348, "ClockID"=w344, "Timestamp Pair"=w339, "Clock History Map in"=w353) -> ("error out"=w349:errorcluster, "Clock History Map out"=w351:map{u8, T41})  [unwired: 4 in]
        n174 = Bundle By Name(cluster=w352, "Clock History Map"=w351) -> (w338:refnum<class "CIFPluginManager.lvclass">)
        n175 = call "Create Error Message.vi"("error in (no error)"=w349) -> ("Error Message"=w350:T31)  [unwired: 3 in]
        n176 = call "Set Manager UpdateClock Response.vi"("Message Data"=w350, "gRPCid in"=w355) -> ("error out"=w354:errorcluster)  [unwired: 9 in]
        n177 = Merge Errors(w349, w354) -> (w357:errorcluster)
      }
      event User Event {
        n178 = event-data() -> ("gRPCid"=w384:T29)  [unwired: 1 in]
        n179 = call "Get Manager CreateOrch Request.vi"("gRPCid"=w384) -> ("error out"=w379:errorcluster, "Message Data"=w378:T44, "gRPCid out"=w383:T29)  [unwired: 8 in]
        n180 = Unbundle By Name(w378) -> ("start_timestamp"=w377:u64, "filename"=w372:string, "default_ip"=w373:string, "orchestration_language"=w368:T45, "create_file"=w367:bool)
        n181 = Not Equal To 0?(x=w377) -> (x != 0?=w376:bool)
        n182 = call <vilib>:"Trim Whitespace.vi"("string"=w372) -> ("trimmed string"=w358:string)  [unwired: 1 in]
        n183 = call <vilib>:"Trim Whitespace.vi"("string"=w373) -> ("trimmed string"=w371:string)  [unwired: 1 in]
        n184 = call "Get Config Log.vi"("Default Timestamp"=w377, "error in (no error)"=w379, "Parse All"=w376, "Plugin Manager in"=w381) -> ("error out"=w374:errorcluster, "Filtered Config Entries"=w375:string, "Plugin Manager out"=w380:refnum<class "CIFPluginManager.lvclass">)  [unwired: 5 in]
        n185 = Empty String/Path?(string/path=w371) -> (empty?=w370:bool)
        n186 = Not(x=w370) -> (.not. x?=w369:bool)
        n187 = case shown="\"PYTHON\", Default" w368 {
          tunnel: w375 -> [w398]
          tunnel: w374 -> [w397]
          tunnel: w358 -> [w396]
          tunnel: w371 -> [w395]
          tunnel: w369 -> [w394]
          tunnel: [w393] -> w365
          tunnel: [w392] -> w366
          tunnel: [w391] -> w359
          frame "PYTHON", Default {
            n188 = call "Create Python Orchestration Script.vi"("Override Address"=w394, "error in"=w397, "Default Address"=w395, "Configuration File Name"=w396, "Filtered Config Entries"=w398) -> ("error out"=w393:errorcluster, "Orchestration File Path"=w392:path, "Python Orchestration File"=w391:string)  [unwired: 4 in]
          }
        }
        n189 = case shown="True" w367 {
          tunnel: w359 -> [_ w388]
          tunnel: w366 -> [_ w389]
          tunnel: w365 -> [w386 w390]
          tunnel: [w386 w387] -> w362
          frame False {
          }
          frame True {
            n190 = Write to Text File(file (use dialog)=w389, text=w388, error in=w390) -> (error out=w387:errorcluster)  [unwired: 1 in, 2 out]
          }
        }
        n191 = call "Create Error Message.vi"("error in (no error)"=w362) -> ("Error Message"=w363:T31)  [unwired: 3 in]
        n192 = Bundle By Name(cluster=T28 {"orchestration_script"="", "status"={"code"=0, "message"=""}} ("Message Data"), "status"=w363) -> (w361:T28)
        n193 = Bundle By Name(cluster=w361, "orchestration_script"=w359) -> (w360:T28)
        n194 = call "Set Manager CreateOrch Response.vi"("Message Data"=w360, "gRPCid in"=w383) -> ("error out"=w382:errorcluster)  [unwired: 9 in]
        n195 = Merge Errors(w362, w382) -> (w385:errorcluster)
      }
      event User Event {
        n196 = event-data() -> ()  [unwired: 1 in, 1 out]
      }
    }
    n197 = Unbundle By Name(w12) -> ("code"=w13:i32)
    n198 = case shown="-1001, 0" w13 {
      tunnel: w12 -> [_ w20]
      frame -1001, 0 {
        # "-1001 is cancelled by client.  Not an error."
      }
      frame 1, Default {
        n199 = call "Write Error.vi"("error in (no error)"=w20, "Plugin Name"="CIF Manager") -> ()  [unwired: 2 in, 1 out]
      }
    }
  }
  n200 = Unbundle By Name(w5) -> ("gRPC Server"=w3:refnum<class "Servicer.lvclass">)
  n201 = Unregister For Events(event registration refnum=w6) -> (error out=w4:errorcluster)  [unwired: 1 in]
  n202 = call <vilib>:"Stop Server.vi"("error in"=w4, "gRPC Server in"=w3) -> ("error out"=w2:errorcluster)  [unwired: 9 in]
  n203 = call "Destroy.vi"("error in (no error)"=w2, "Plugin Manager in"=w5) -> ("error out"=→"error out":errorcluster)  [unwired: 8 in, 1 out]
